vi "数据查询筛选弹框.vi"(8 "error in (no error)":errorcluster caption="错误输入（无错误）", 9 "是否初始化":enum16{"init", "keep"}(ring), 10 "database":string="database1.mdb", 11 "table":string(combo)="CODMn") -> (0 "error out":errorcluster caption="错误输出", 1 "确定输出":bool, 2 "显示项":string[](array[string]), 3 "condition":string)   [LabVIEW 2016]
uses:
  <vilib>/addons/database/Auxilliary.llb/DB Tools DataTypes.ctl
  <vilib>/picture/picture.llb/imagedata.ctl
  <vilib>/Utility/miscctls.llb/LVPointTypeDef.ctl
  <vilib>/addons/database/Connection.llb/DB Tools Open Connec (String).vi
  <vilib>/addons/database/Connection.llb/Conn Execute.vi
  <vilib>/addons/database/Recordset.llb/Rec Fetch Recordset Data (R).vi
  <vilib>/addons/database/Recordset.llb/Rec Destroy - Connection.vi
  <userlib>/_OpenG.lib/array/array.llb/Remove Duplicates from 1D Array (String)__ogtk.vi
  <vilib>/addons/database/_DB Variant To Data/Database Variant To Data.xnode
  <vilib>/addons/database/NI_Database_API.lvlib
panel:
  in  "背景图像":T1
  in  "实时分钟小时数据":enum32{"实时数据", "分钟数据", "小时数据"}(radio)
  in  "确定":bool
  out "自定义2single":cluster{"起始范围":string, "截止范围":string}
  out "自定义1single":cluster{"起始范围":string, "截止范围":string}
  out "自定义2筛选条件":string[](array[string])
  out "自定义1筛选条件":string[](array[string])
  in  "标签 2":string="从：\n\n\n至："
  in  "自定义数值结束 2":dbl
  in  "自定义数值起始 2":dbl
  in  "自定义结束时间 2":timestamp(xcontrol)
  in  "自定义起始时间 2":timestamp(xcontrol)
  in  "自定义 2":T2 caption="自定义"
  in  "下拉列表":string(xcontrol)
  in  "标签":string="从：\n\n\n至："
  in  "自定义数值结束":dbl
  in  "自定义数值起始":dbl
  in  "自定义结束时间":timestamp(xcontrol)
  in  "自定义起始时间":timestamp(xcontrol)
  in  "自定义":T2
  in  "下拉列表 2":string(xcontrol)
  out "type":T3[](array[typedef])
  out "所有测量模式":string[](array[string])
  out "数组":string[](array[string])
  out "columns":string[](array[string])
  in  "测量模式":T4
  in  "退出":bool
  in  "清空":bool
  in  "时间标识输入1":timestamp(xcontrol)
  in  "时间标识输入2":timestamp(xcontrol)
  # "时间"
  # "从："
  # "至："
  # "测试模式"
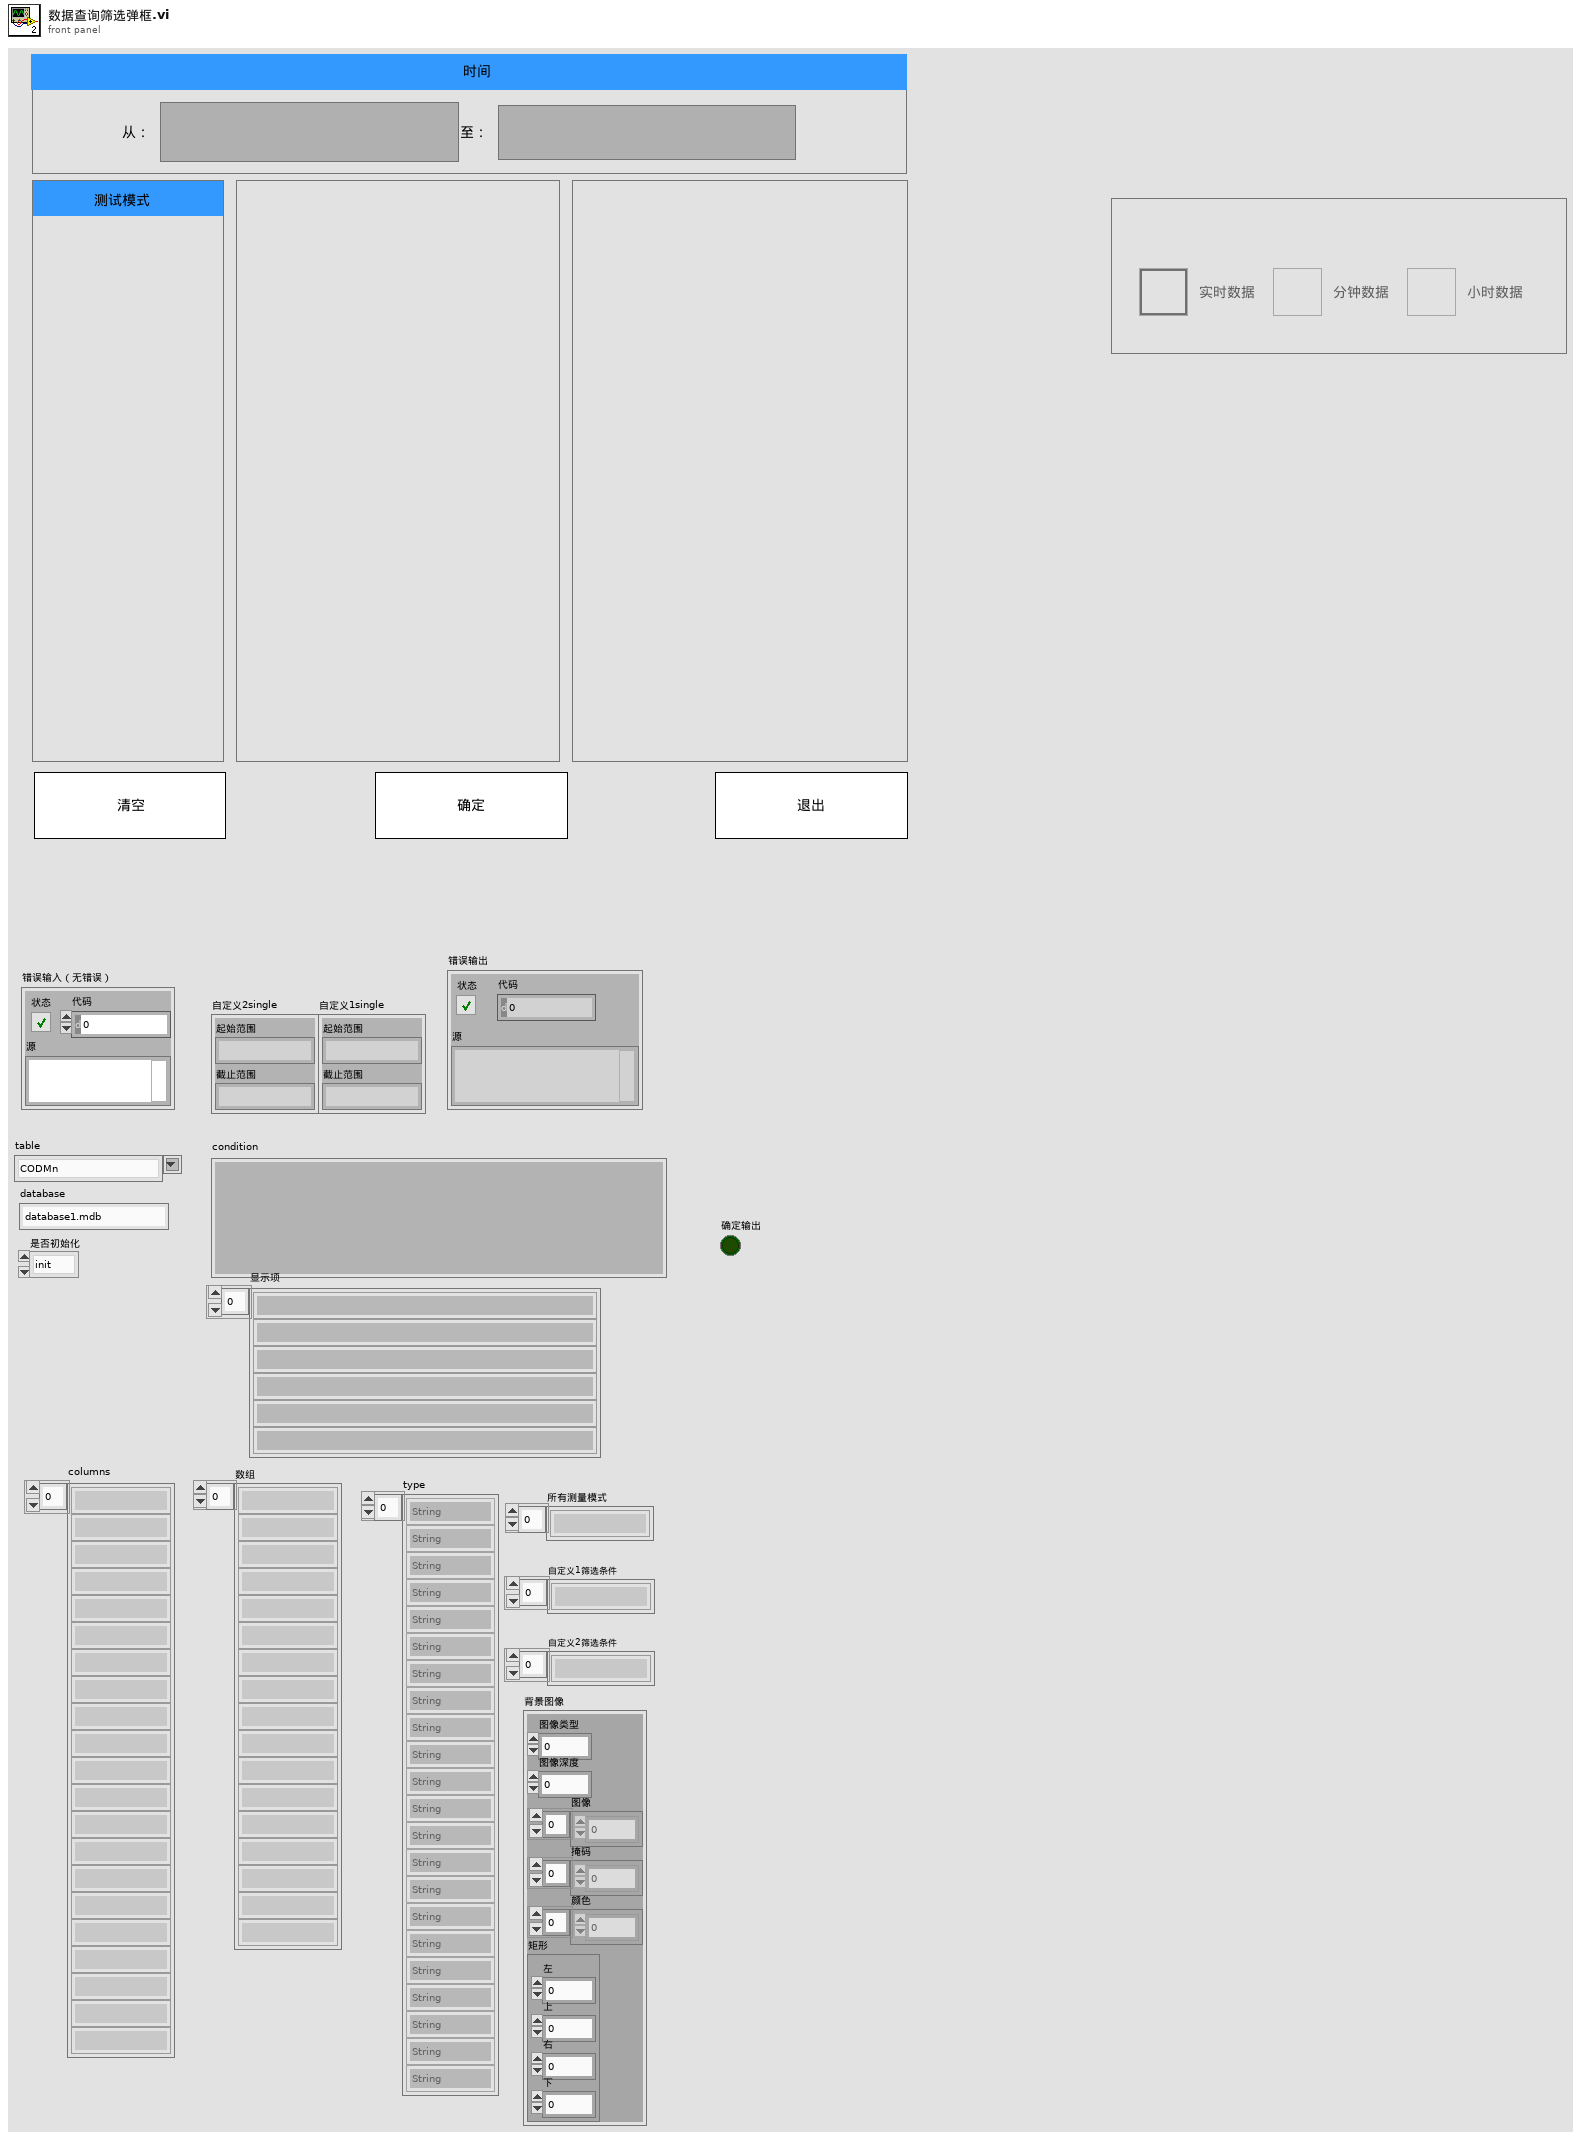
[diagram p1: front panel]
types:
  T1 = typedef "imagedata.ctl" = cluster{"image type":i32, "image depth":i32, "image":u8[], "mask":u8[], "colors":u32[], "Rectangle":cluster{"left":i16, "top":i16, "right":i16, "bottom":i16}}
  T2 = cluster{"DSADSA ":bool, "2":bool, "3":bool, "4":bool, "5":bool, "6":bool, "7":bool, "8":bool, "9":bool, "10":bool}
  T3 = typedef "NI_Database_API.lvlib/DB Tools DataTypes.ctl" = enum16{"String", "Long (I32)", "Single (SGL)", "Double (DBL)", "Date/Time", "Binary"}
  T4 = cluster{"水样测试":bool, "标样核查":bool, "零点核查":bool, "跨度核查":bool, "空白测试":bool, "平行样测试":bool, "加标回收":bool, "空白校准":bool, "标样校准":bool, "初始化清洗":bool}
  T5 = enum8{"Enabled", "Disabled", "Disabled and Grayed Out"}
  T6 = typedef "LVPointTypeDef.ctl" = cluster{"Horizontal":i16, "Vertical":i16}
  T7 = typedef "NI_Database_API.lvlib/Conn ObjectReference.ctl" = refnum<k1>
  T8 = cluster{"name":string, "database data type":T3, "defined size":i32}[]
  T9 = typedef "NI_Database_API.lvlib/Rec ObjectReference.ctl" = refnum<k1>
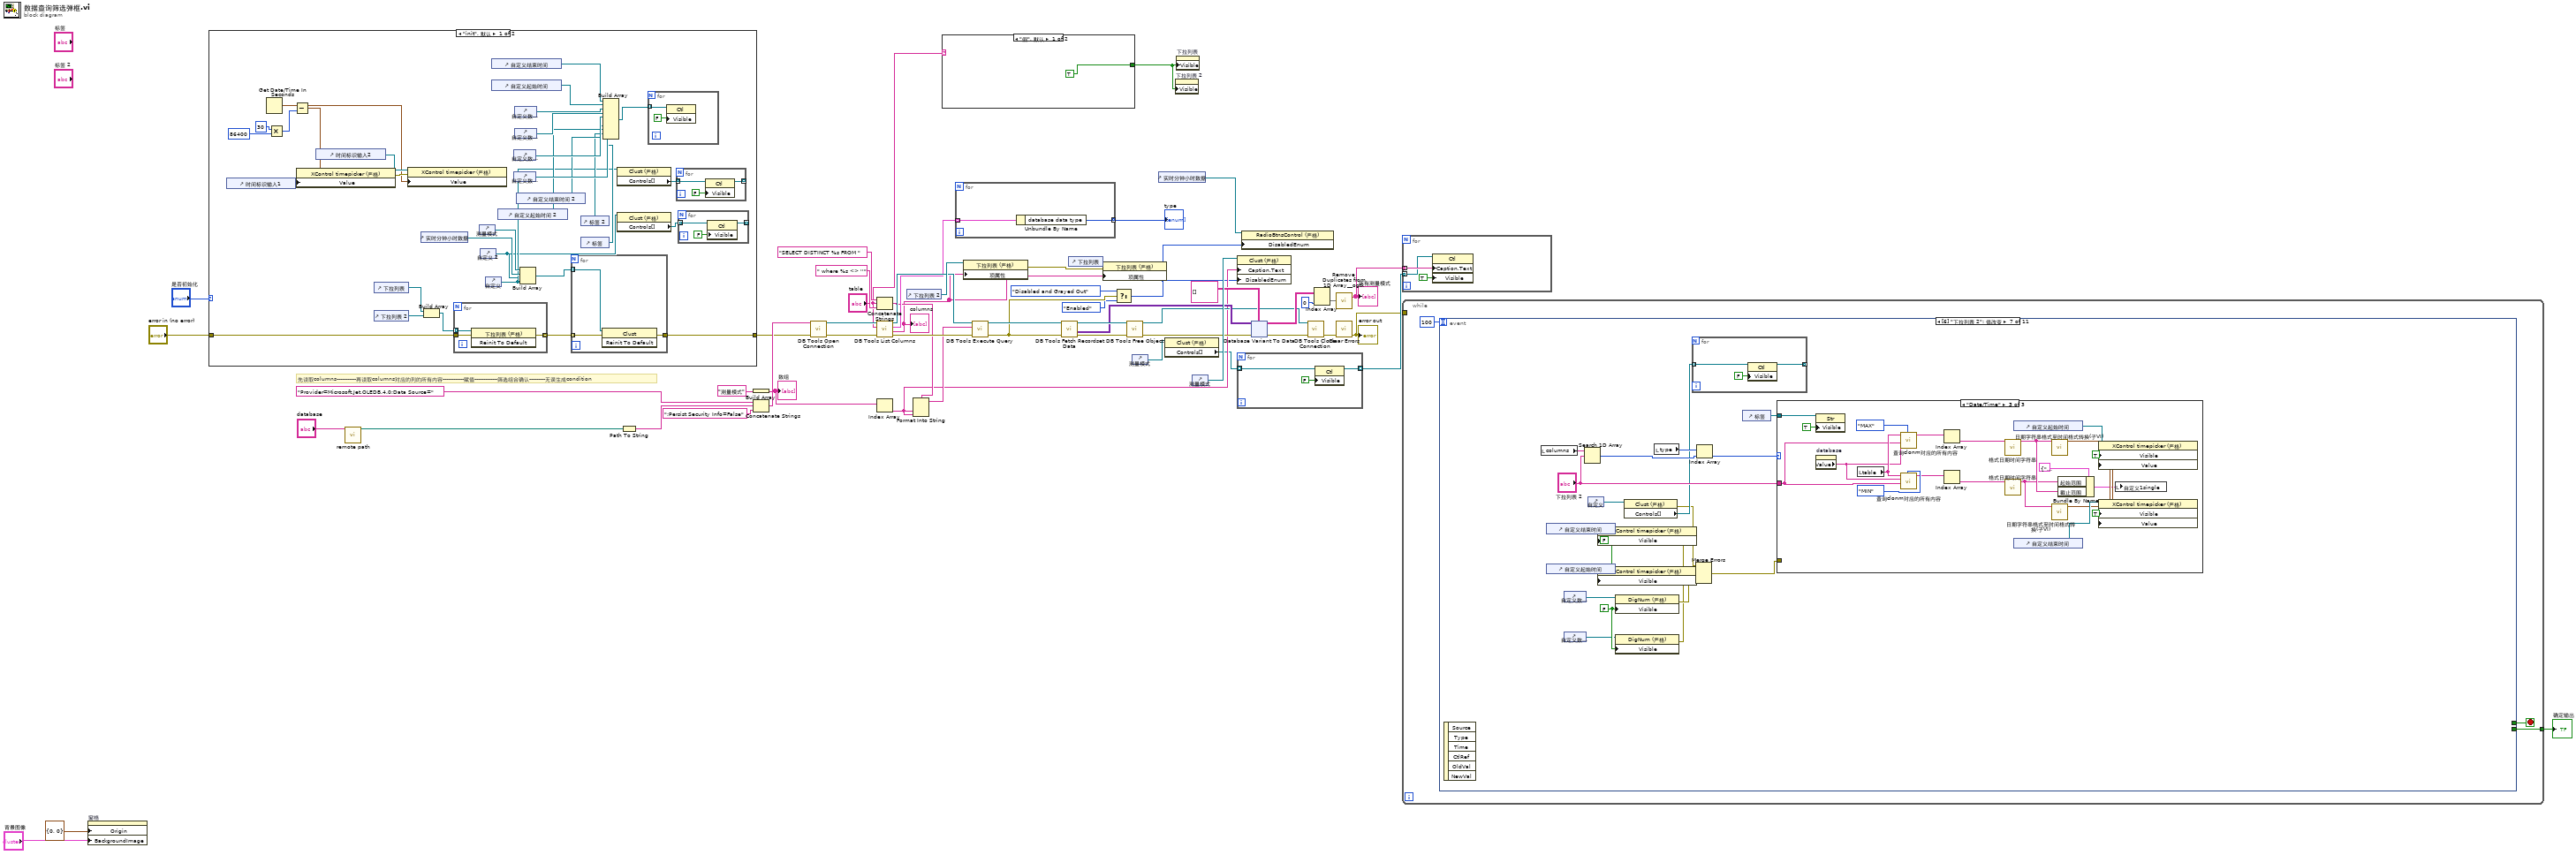
[diagram p0: block diagram]
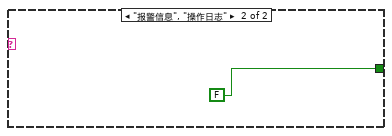
[diagram p2: hidden frame]
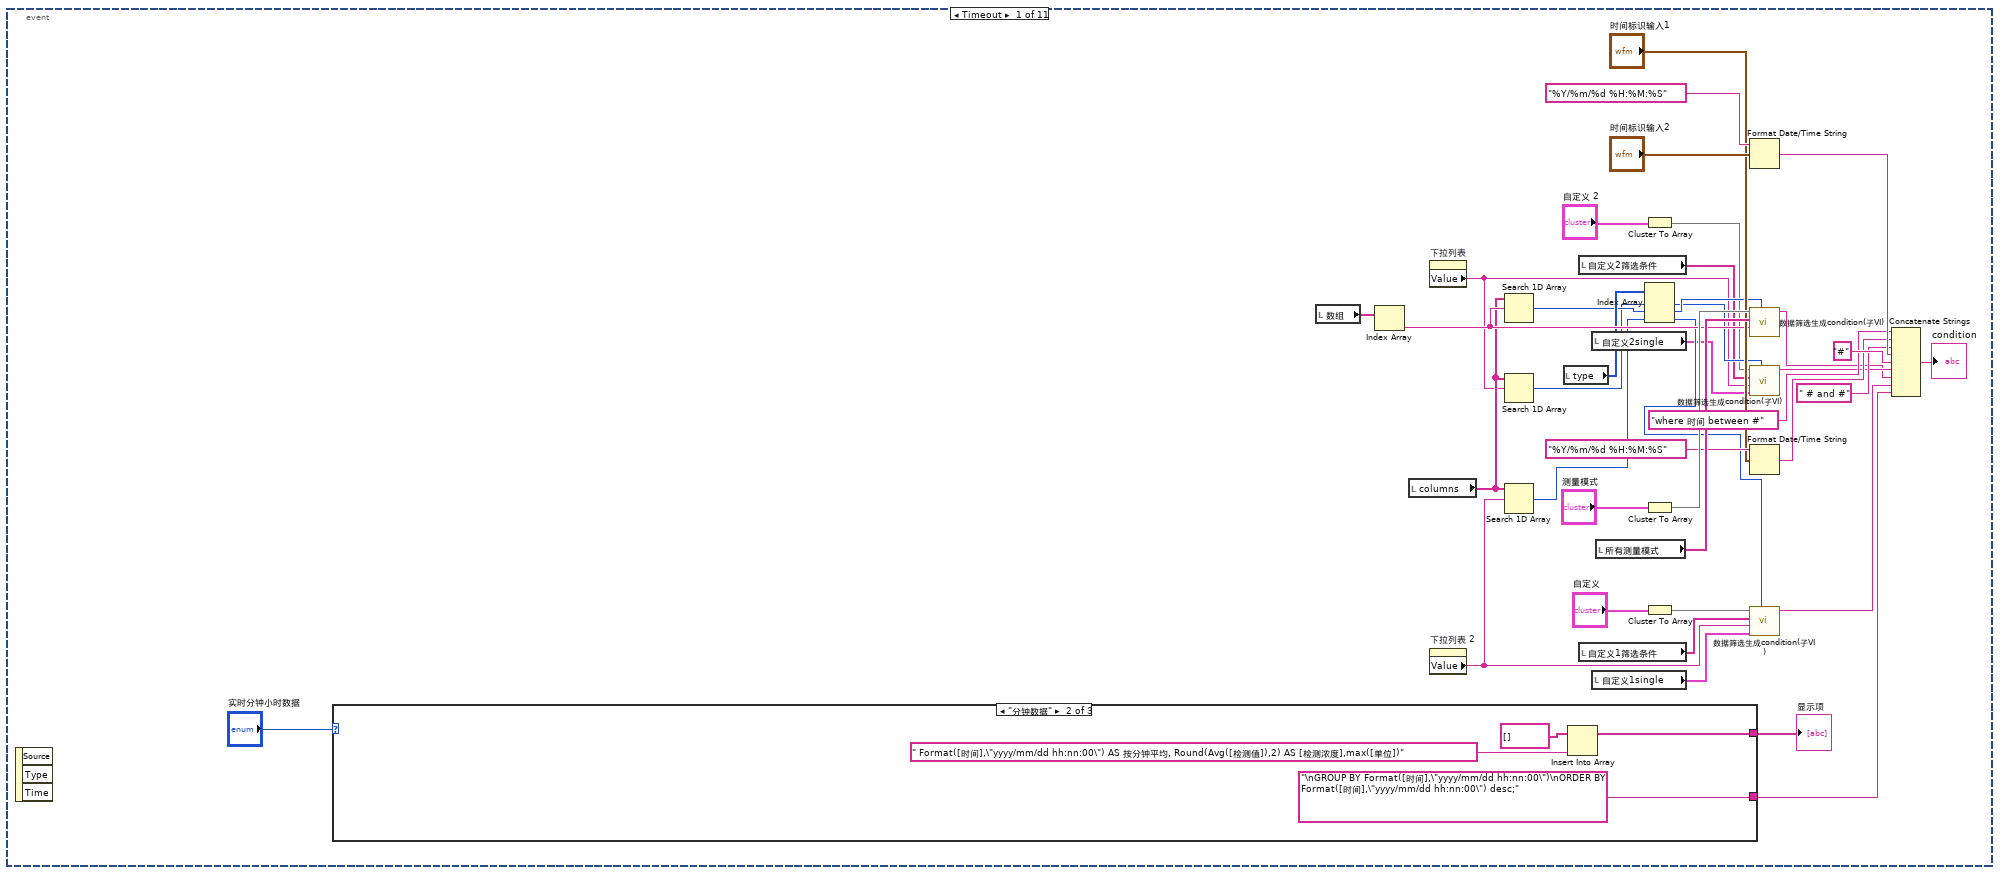
[diagram p4: hidden frame]
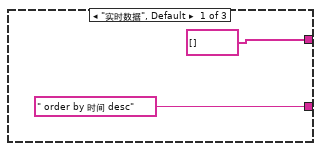
[diagram p5: hidden frame]
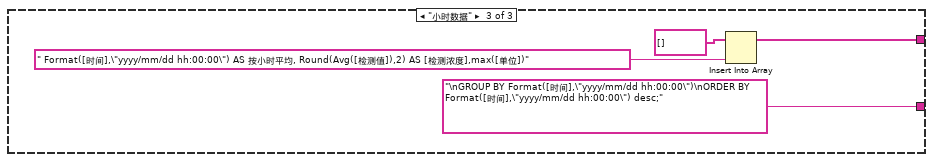
[diagram p6: hidden frame]
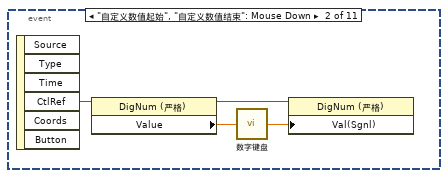
[diagram p7: hidden frame]
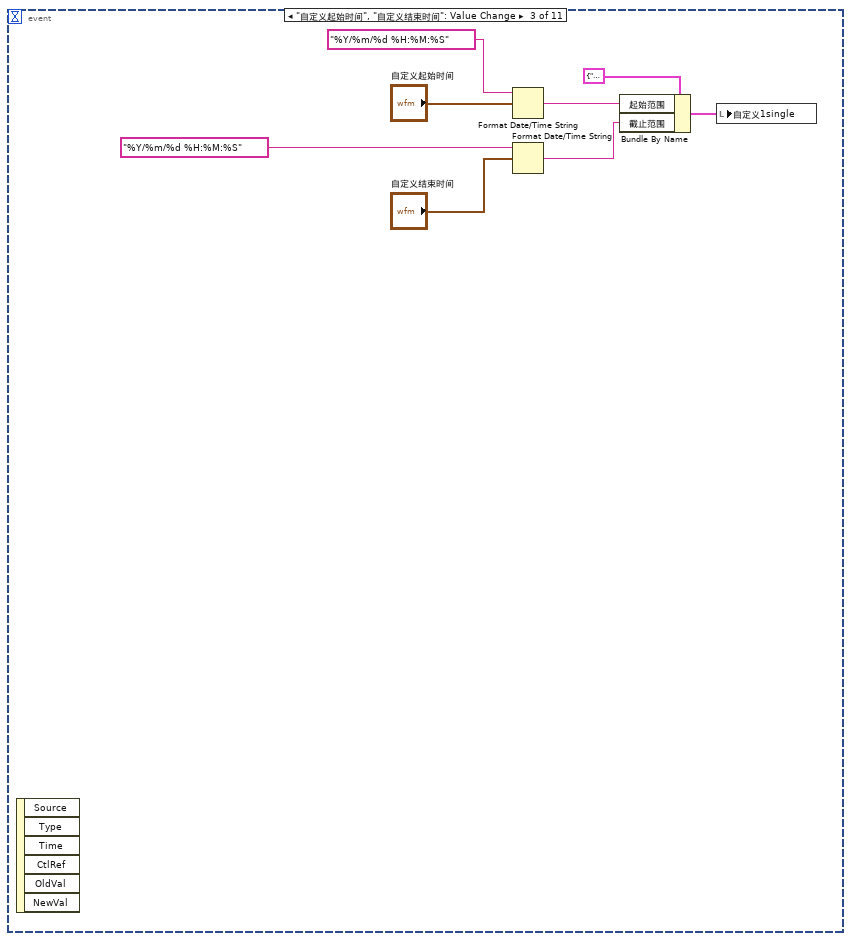
[diagram p8: hidden frame]
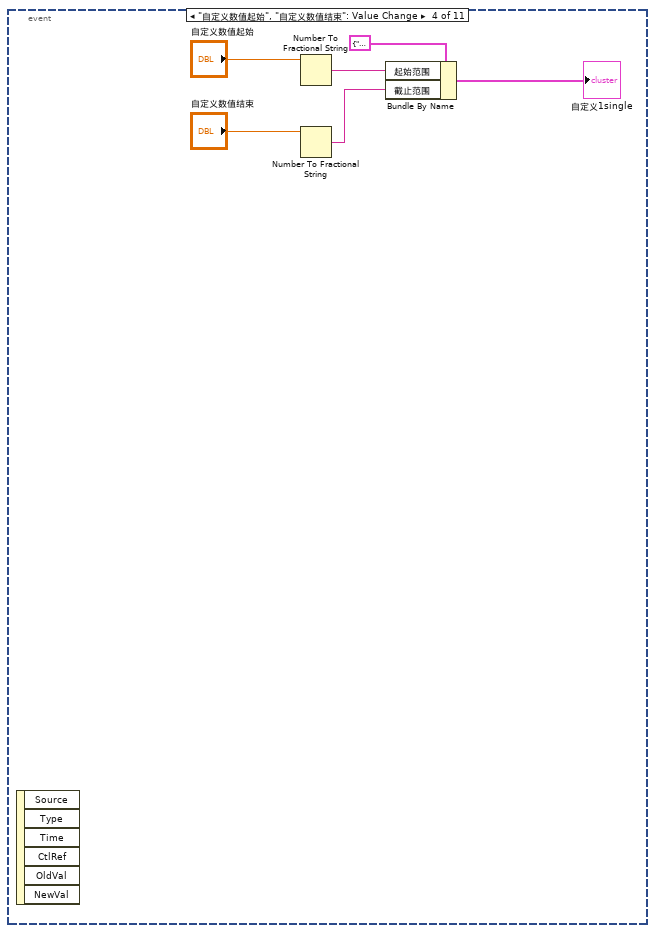
[diagram p9: hidden frame]
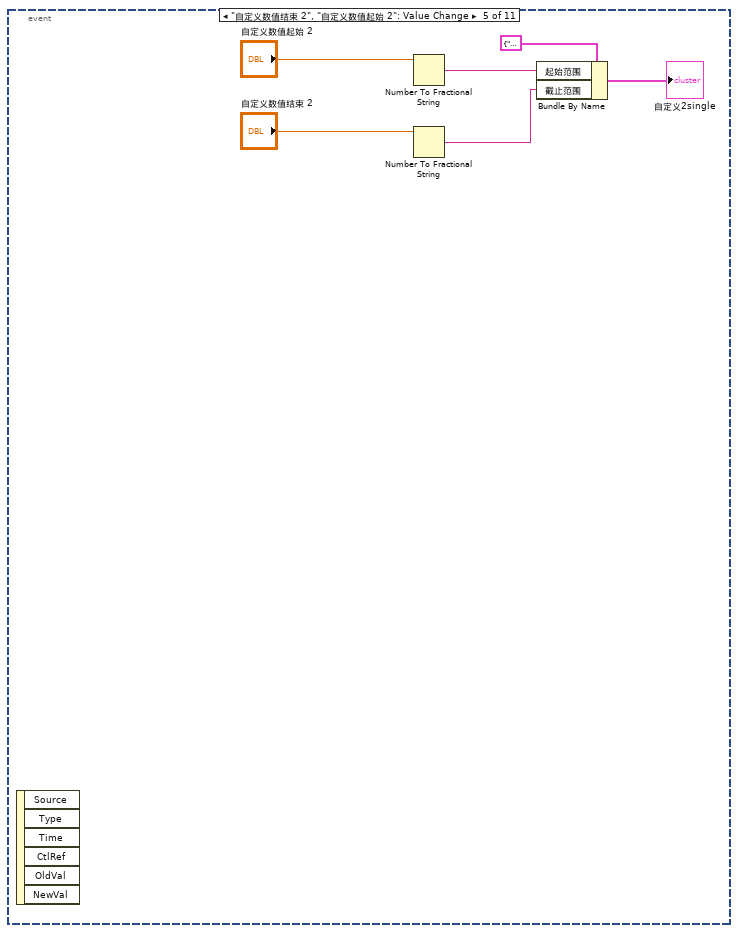
[diagram p10: hidden frame]
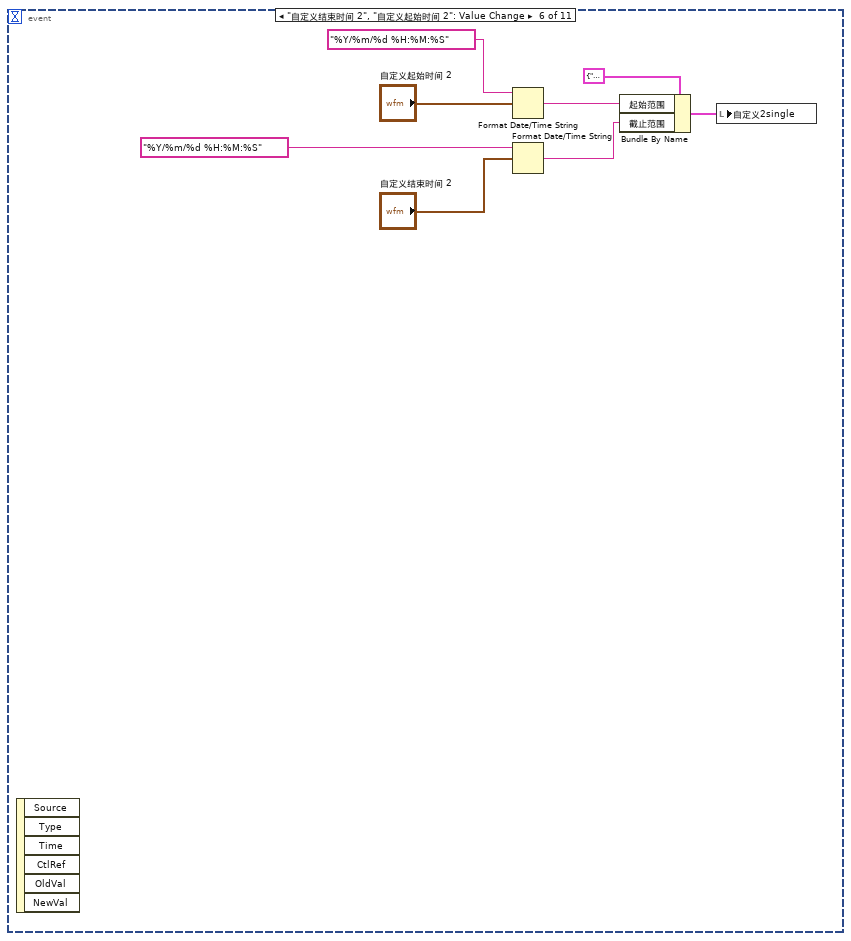
[diagram p11: hidden frame]
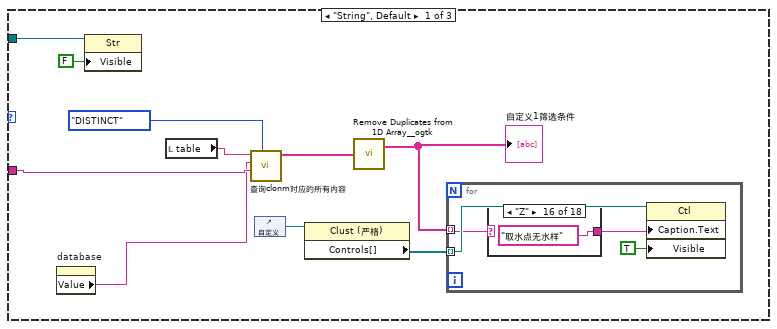
[diagram p12: hidden frame]
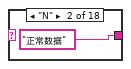
[diagram p14: hidden frame]
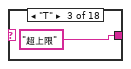
[diagram p15: hidden frame]
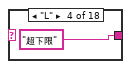
[diagram p16: hidden frame]
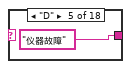
[diagram p17: hidden frame]
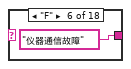
[diagram p18: hidden frame]
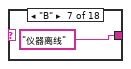
[diagram p19: hidden frame]
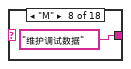
[diagram p20: hidden frame]
diagram:
  # "先读取columns-----------再读取columns对应的列的所有内容------------赋值-------------筛选组合确认---------无误生成condition"
  n1 = property on="窗格" class="Pane"("Origin"=T6 {"Horizontal"=0, "Vertical"=0} ("原点"), "BackgroundImage"="背景图像") -> ()  [unwired: 2 in, 2 out]
  n2 = case shown="\"init\", 默认" "是否初始化" {
    tunnel: "error in (no error)" -> [w64 w101]
    tunnel: [w83 w101] -> w11
    frame "init", Default {
      n3 = control-ref of="时间标识输入1"() -> (w66:refnum<vi>)
      n4 = Get Date/Time In Seconds() -> (seconds since 1Jan1904=w59:timestamp)
      n5 = Multiply(x=30, y=86400) -> (x*y=w78:i32)
      n6 = Subtract(x=w59, y=w78) -> (x-y=w82:timestamp)
      n7 = property class="XControl timepicker (严格)"(reference=w66, "Value"=w82) -> (error out=w81:errorcluster)  [unwired: 1 in, 1 out]
      n8 = control-ref of="时间标识输入2"() -> (w65:refnum<vi>)
      n9 = control-ref of="下拉列表"() -> (w62:refnum<vi>)
      n10 = control-ref of="下拉列表 2"() -> (w61:refnum<vi>)
      n11 = property class="XControl timepicker (严格)"(reference=w65, error in=w81, "Value"=w59) -> ()  [unwired: 2 out]
      n12 = control-ref of="实时分钟小时数据"() -> (w86:refnum<vi>)
      n13 = Build Array(w62, w61) -> (w60:refnum<vi>[])
      n14 = for {
        tunnel: w64 -> [w95]
        tunnel: [w94] -> w63 mode=indexing
        tunnel: w60 -> [w93] mode=indexing
        n15 = invoke class="下拉列表 (严格)" method="Reinit To Default"(reference=w93, error in=w95) -> (error out=w94:errorcluster)  [unwired: 1 in, 2 out]
      }
      n16 = control-ref of="测量模式"() -> (w84:refnum<vi>)
      n17 = control-ref of="自定义 2"() -> (w56:refnum<vi>)
      n18 = control-ref of="自定义"() -> (w58:refnum<vi>)
      n19 = control-ref of="自定义结束时间"() -> (w77:refnum<vi>)
      n20 = control-ref of="自定义起始时间"() -> (w76:refnum<vi>)
      n21 = control-ref of="自定义起始时间 2"() -> (w71:refnum<vi>)
      n22 = control-ref of="自定义数值结束 2"() -> (w73:refnum<vi>)
      n23 = control-ref of="自定义数值起始 2"() -> (w72:refnum<vi>)
      n24 = control-ref of="自定义数值结束"() -> (w75:refnum<vi>)
      n25 = control-ref of="自定义数值起始"() -> (w74:refnum<vi>)
      n26 = control-ref of="自定义结束时间 2"() -> (w70:refnum<vi>)
      n27 = Build Array(w84, w86, w56, w58) -> (w85:refnum<vi>[])
      n28 = for {
        tunnel: w85 -> [w100] mode=indexing
        tunnel: w63 -> [w99] mode=indexing
        tunnel: [w98] -> w83
        n29 = invoke class="Clust" method="Reinit To Default"(reference=w100, error in=w99) -> (error out=w98:errorcluster)  [unwired: 1 in, 2 out]
      }
      n30 = control-ref of="标签 2"() -> (w67:refnum<vi>)
      n31 = control-ref of="标签"() -> (w68:refnum<vi>)
      n32 = Build Array(w77, w76, w75, w74, w73, w72, w70, w71, w67, w68) -> (w69:refnum<vi>[])
      n33 = property class="Clust (严格)"(reference=w58) -> ("Controls[]"=w57:refnum<vi>[])  [unwired: 1 in, 2 out]
      n34 = property class="Clust (严格)"(reference=w56) -> ("Controls[]"=w55:refnum<vi>[])  [unwired: 1 in, 2 out]
      n35 = for {
        tunnel: w69 -> [w97] mode=indexing
        n36 = property class="Ctl"(reference=w97, "Visible"=FALSE ("可见")) -> ()  [unwired: 1 in, 2 out]
      }
      n37 = for {
        tunnel: w57 -> [w92] mode=indexing
        tunnel: [w90] -> _ mode=indexing
        n38 = property class="Ctl"(reference=w92, "Visible"=FALSE ("可见")) -> (reference out=w90:refnum<vi>)  [unwired: 1 in, 1 out]
      }
      n39 = for {
        tunnel: w55 -> [w89] mode=indexing
        tunnel: [w87] -> _ mode=indexing
        n40 = property class="Ctl"(reference=w89, "Visible"=FALSE ("可见")) -> (reference out=w87:refnum<vi>)  [unwired: 1 in, 1 out]
      }
    }
    frame "keep" {
    }
  }
  n41 = call "remote path.vi"("database"="database") -> ("appended path"=w49:path)  [unwired: 10 in]
  n42 = Path To String(path=w49) -> (string=w51:string)
  n43 = Build Array("测量模式" ("Element Data")) -> (w14:string[])
  "数组" <- w14
  n44 = Concatenate Strings("Provider=Microsoft.Jet.OLEDB.4.0;Data Source=", w51, ";Persist Security Info=False") -> (w50:string)
  n45 = call-poly <vilib>:"DB Tools Open Connection.vi"("error in (no error)"=w11, "connection information"=w50) -> ("error out"=w47:errorcluster, "connection reference"=w48:T7)  [unwired: 6 in]
  n46 = Concatenate Strings("SELECT DISTINCT %s FROM " ("字符串"), "table", " where %s <> ''" ("字符串")) -> (w24:string)
  n47 = call <vilib>:"DB Tools List Columns.vi"("error in (no error)"=w47, "table"="table", "connection reference"=w48) -> ("error out"=w41:errorcluster, "columns"=w4:string[], "column information"=w28:T8, "connection reference out"=w29:T7)  [unwired: 1 in]
  "columns" <- w4
  n48 = Index Array(array=w14) -> (element=w23:string)  [unwired: 1 in]
  n49 = control-ref of="下拉列表 2"() -> (w30:refnum<vi>)
  n50 = Format Into String(format string=w24, w23, w23) -> (resulting string=w40:string)  [unwired: 2 in, 1 out]
  n51 = case shown="\"假\", 默认" "table" {
    tunnel: [TRUE FALSE] -> w1
    frame "假", Default {
    }
    frame "报警信息", "操作日志" {
    }
  }
  n52 = for {
    tunnel: w28 -> [w105] mode=indexing
    tunnel: [w104] -> w27 mode=indexing
    n53 = Unbundle By Name(w105) -> ("database data type"=w104:T3)
  }
  "type" <- w27
  n54 = property class="下拉列表 (严格)"(reference=w30, "项属性"=w4) -> (error out=w10:errorcluster)  [unwired: 1 in, 1 out]
  n55 = call-poly <vilib>:"DB Tools Execute Query.vi"("error in (no error)"=w41, "SQL query"=w40, "connection reference"=w29) -> ("error out"=w22:errorcluster, "recordset reference"=w44:T9)  [unwired: 5 in]
  n56 = call-poly <vilib>:"DB Tools Fetch Recordset Data.vi"("error in (no error)"=w22, "recordset reference"=w44) -> ("error out"=w43:errorcluster, "recordset data"=w36:variant[][], "recordset reference out"=w42:T9)  [unwired: 3 in]
  n57 = control-ref of="下拉列表"() -> (w19:refnum<vi>)
  n58 = property class="下拉列表 (严格)"(reference=w19, error in=w10, "项属性"=w4) -> ()  [unwired: 2 out]
  n59 = Select(t=T5."Disabled and Grayed Out" ("禁用"), s=w22, f=T5."Enabled" ("禁用")) -> (s? t:f=w6:T5)
  n60 = call-poly <vilib>:"DB Tools Free Object.vi"("error in (no error)"=w43, "recordset reference"=w42) -> ("error out"=w35:errorcluster, "connection reference"=w34:T7)  [unwired: 8 in]
  n61 = control-ref of="测量模式"() -> (w54:refnum<vi>)
  n62 = control-ref of="实时分钟小时数据"() -> (w7:refnum<vi>)
  n63 = property class="Clust (严格)"(reference=w54) -> ("Controls[]"=w18:refnum<vi>[])  [unwired: 1 in, 2 out]
  n64 = property on="下拉列表 2" class="下拉列表 (严格)"("Visible"=w1) -> ()  [unwired: 2 in, 2 out]
  n65 = property on="下拉列表" class="下拉列表 (严格)"("Visible"=w1) -> ()  [unwired: 2 in, 2 out]
  n66 = control-ref of="测量模式"() -> (w45:refnum<vi>)
  n67 = property class="Clust (严格)"(reference=w45, "Caption.Text"=w23, "DisabledEnum"=w6) -> ()  [unwired: 1 in, 2 out]
  n68 = for {
    tunnel: w18 -> [w108] mode=indexing
    tunnel: [w106] -> w17 mode=indexing
    n69 = property class="Ctl"(reference=w108, "Visible"=FALSE ("可见")) -> (reference out=w106:refnum<vi>)  [unwired: 1 in, 1 out]
  }
  n70 = property class="RadioBtnsControl (严格)"(reference=w7, "DisabledEnum"=w6) -> ()  [unwired: 1 in, 2 out]
  n71 = xnode "Database Variant To Data"("database variant"=w36, "error in (no error)"=w35, "type"=string[][] []) -> ("data"=w37:string[][], "error out"=w38:errorcluster)
  n72 = call <vilib>:"DB Tools Close Connection.vi"("error in (no error)"=w38, "connection reference"=w34) -> ("error out"=w13:errorcluster)  [unwired: 5 in]
  n73 = Index Array(array=w37, index (col)=0 ("禁用的索引 (列)")) -> (element=w32:string[])  [unwired: 1 in]
  n74 = call-poly <userlib>:"Remove Duplicates from 1D Array__ogtk.vi"("Input Array"=w32) -> ("Output Array"=w16:string[])  [unwired: 1 out]
  "所有测量模式" <- w16
  n75 = call <vilib>:"Clear Errors.vi"("error in (no error)"=w13) -> ("error out"=w8:errorcluster)  [unwired: 5 in, 1 out]
  "error out" <- w8
  n76 = for {
    tunnel: w16 -> [w111] mode=indexing
    tunnel: w17 -> [w109] mode=indexing
    n77 = property class="Ctl"(reference=w109, "Caption.Text"=w111, "Visible"=TRUE ("可见")) -> ()  [unwired: 1 in, 2 out]
  }
  n78 = while {
    tunnel: [w112] -> w15
    tunnel: w8 -> [_]
    stop <- w114 stop-if-true
    n79 = event shown="[6] \"下拉列表 2\": 值改变" {
      selector: _ -> [_ _ _ _ _ _ _ _ _ _ _]
      dyn-events: _ -> [_ _ _ _ _ _ _ _ _ _ _]
      timeout: 100 -> [_ _ _ _ _ _ _ _ _ _ _]
      tunnel: [_ _ _ _ _ _ _ _ _ w394 TRUE] -> w114
      tunnel: [_ _ _ _ _ _ _ _ _ w394 _] -> w112
      event Timeout {
        n80 = event-data() -> ()  [unwired: 1 in, 3 out]
        n81 = case shown="\"分钟数据\"" "实时分钟小时数据" {
          tunnel: [string[] [] ("显示项") w156 w160] -> w115
          tunnel: [" order by 时间 desc" ("字符串") "\nGROUP BY Format([时间],\"yyyy/mm/dd hh:nn:00\")\nORDER BY Format([时间],\"yyyy/mm/dd hh:nn:00\") desc;" ("字符串") "\nGROUP BY Format([时间],\"yyyy/mm/dd hh:00:00\")\nORDER BY Format([时间],\"yyyy/mm/dd hh:00:00\") desc;" ("字符串")] -> w116
          frame "实时数据", Default {
          }
          frame "分钟数据" {
            n82 = Insert Into Array(array=string[] [] ("显示项"), new element=" Format([时间],\"yyyy/mm/dd hh:nn:00\") AS 按分钟平均, Round(Avg([检测值]),2) AS [检测浓度],max([单位])" ("新元素/子数组")) -> (w156:string[])  [unwired: 1 in]
          }
          frame "小时数据" {
            n83 = Insert Into Array(array=string[] [] ("显示项"), new element=" Format([时间],\"yyyy/mm/dd hh:00:00\") AS 按小时平均, Round(Avg([检测值]),2) AS [检测浓度],max([单位])" ("新元素/子数组")) -> (w160:string[])  [unwired: 1 in]
          }
        }
        "显示项" <- w115
        n84 = local read "数组"() -> (w153:string[])
        n85 = Index Array(array=w153) -> (element=w139:string)  [unwired: 1 in]
        n86 = local read "columns"() -> (w133:string[])
        n87 = property on="下拉列表" class="下拉列表 (严格)"() -> ("Value"=w124:string)  [unwired: 2 in, 2 out]
        n88 = property on="下拉列表 2" class="下拉列表 (严格)"() -> ("Value"=w123:string)  [unwired: 2 in, 2 out]
        n89 = Search 1D Array(1D array=w133, element=w139) -> (index of element=w137:i32)  [unwired: 1 in]
        n90 = Search 1D Array(1D array=w133, element=w124) -> (index of element=w132:i32)  [unwired: 1 in]
        n91 = Search 1D Array(1D array=w133, element=w123) -> (index of element=w135:i32)  [unwired: 1 in]
        n92 = local read "type"() -> (w138:T3[])
        n93 = local read "自定义2筛选条件"() -> (w121:string[])
        n94 = local read "自定义1筛选条件"() -> (w122:string[])
        n95 = local read "自定义2single"() -> (w119:cluster{"起始范围":string, "截止范围":string})
        n96 = local read "自定义1single"() -> (w118:cluster{"起始范围":string, "截止范围":string})
        n97 = local read "所有测量模式"() -> (w152:string[])
        n98 = Cluster To Array(cluster="自定义 2") -> (array=w130:bool[])
        n99 = Index Array(array=w138, index #1=w132, index #2=w137, index #3=w135) -> (element #1=w131:T3, element #2=w136:T3, element #3=w134:T3)
        n100 = Cluster To Array(cluster="测量模式") -> (array=w151:bool[])
        n101 = Cluster To Array(cluster="自定义") -> (array=w120:bool[])
        n102 = Format Date/Time String(time format string (%c)="%Y/%m/%d %H:%M:%S" ("时间格式字符串(%c)"), seconds (now)="时间标识输入2") -> (date/time string=w148:string)  [unwired: 1 in]
        n103 = call "数据筛选生成condition(子VI).vi"("database data type"=w136, "段名"=w139, "筛选内容"=w152, "簇转数组"=w151) -> ("condition"=w128:string)  [unwired: 7 in]
        n104 = call "数据筛选生成condition(子VI).vi"("database data type"=w131, "Single"=w119, "段名"=w124, "筛选内容"=w121, "簇转数组"=w130) -> ("condition"=w129:string)  [unwired: 6 in]
        n105 = Format Date/Time String(time format string (%c)="%Y/%m/%d %H:%M:%S" ("时间格式字符串(%c)"), seconds (now)="时间标识输入1") -> (date/time string=w146:string)  [unwired: 1 in]
        n106 = call "数据筛选生成condition(子VI).vi"("database data type"=w134, "Single"=w118, "段名"=w123, "筛选内容"=w122, "簇转数组"=w120) -> ("condition"=w127:string)  [unwired: 6 in]
        n107 = Concatenate Strings("where 时间 between #", w146, " # and #" ("condition"), w148, "#" ("condition"), w129, w128, w127, w116) -> (→"condition":string)
      }
      event "自定义数值起始", "自定义数值结束": Mouse Down {
        n108 = event-data() -> ("CtlRef"=w167:refnum<vi>)  [unwired: 1 in, 5 out]
        n109 = property class="DigNum (严格)"(reference=w167) -> (reference out=w165:refnum<vi>, "Value"=w166:dbl)  [unwired: 1 in, 1 out]
        n110 = call "数字键盘.vi"("OldNumber"=w166) -> ("NewNumber"=w164:sgl)
        n111 = property class="DigNum (严格)"(reference=w165, "Val(Sgnl)"=w164) -> ()  [unwired: 1 in, 2 out]
      }
      event "自定义起始时间", "自定义结束时间": Value Change {
        n112 = event-data() -> ()  [unwired: 1 in, 6 out]
        n113 = Format Date/Time String(time format string (%c)="%Y/%m/%d %H:%M:%S" ("时间格式字符串(%c)"), seconds (now)="自定义起始时间") -> (date/time string=w174:string)  [unwired: 1 in]
        n114 = Format Date/Time String(time format string (%c)="%Y/%m/%d %H:%M:%S" ("时间格式字符串(%c)"), seconds (now)="自定义结束时间") -> (date/time string=w175:string)  [unwired: 1 in]
        n115 = Bundle By Name(cluster=cluster{"起始范围":string, "截止范围":string} {"起始范围"="2", "截止范围"="5"} ("Single"), "起始范围"=w174, "截止范围"=w175) -> (w168:cluster{"起始范围":string, "截止范围":string})
        n116 = local write "自定义1single"(w168) -> ()
      }
      event "自定义数值起始", "自定义数值结束": Value Change {
        n117 = event-data() -> ()  [unwired: 1 in, 6 out]
        n118 = Number To Fractional String(number="自定义数值起始") -> (F-format string=w180:string)  [unwired: 3 in]
        n119 = Number To Fractional String(number="自定义数值结束") -> (F-format string=w181:string)  [unwired: 3 in]
        n120 = Bundle By Name(cluster=cluster{"起始范围":string, "截止范围":string} {"起始范围"="2", "截止范围"="5"} ("Single"), "起始范围"=w180, "截止范围"=w181) -> (→"自定义1single":cluster{"起始范围":string, "截止范围":string})
      }
      event "自定义数值结束 2", "自定义数值起始 2": Value Change {
        n121 = event-data() -> ()  [unwired: 1 in, 6 out]
        n122 = Number To Fractional String(number="自定义数值起始 2") -> (F-format string=w184:string)  [unwired: 3 in]
        n123 = Number To Fractional String(number="自定义数值结束 2") -> (F-format string=w183:string)  [unwired: 3 in]
        n124 = Bundle By Name(cluster=cluster{"起始范围":string, "截止范围":string} {"起始范围"="2", "截止范围"="5"} ("Single"), "起始范围"=w184, "截止范围"=w183) -> (→"自定义2single":cluster{"起始范围":string, "截止范围":string})
      }
      event "自定义结束时间 2", "自定义起始时间 2": Value Change {
        n125 = event-data() -> ()  [unwired: 1 in, 6 out]
        n126 = Format Date/Time String(time format string (%c)="%Y/%m/%d %H:%M:%S" ("时间格式字符串(%c)"), seconds (now)="自定义起始时间 2") -> (date/time string=w193:string)  [unwired: 1 in]
        n127 = Format Date/Time String(time format string (%c)="%Y/%m/%d %H:%M:%S" ("时间格式字符串(%c)"), seconds (now)="自定义结束时间 2") -> (date/time string=w194:string)  [unwired: 1 in]
        n128 = Bundle By Name(cluster=cluster{"起始范围":string, "截止范围":string} {"起始范围"="2", "截止范围"="5"} ("Single"), "起始范围"=w193, "截止范围"=w194) -> (w195:cluster{"起始范围":string, "截止范围":string})
        n129 = local write "自定义2single"(w195) -> ()
      }
      event "下拉列表 2": Value Change {
        w206 = FALSE ("可见")
        w196 = FALSE ("可见")
        n130 = event-data() -> ()  [unwired: 1 in, 6 out]
        n131 = local read "columns"() -> (w213:string[])
        n132 = control-ref of="自定义结束时间"() -> (w208:refnum<vi>)
        n133 = control-ref of="自定义起始时间"() -> (w207:refnum<vi>)
        n134 = control-ref of="自定义数值结束"() -> (w205:refnum<vi>)
        n135 = control-ref of="自定义数值起始"() -> (w198:refnum<vi>)
        n136 = Search 1D Array(1D array=w213, element="下拉列表 2") -> (index of element=w215:i32)  [unwired: 1 in]
        n137 = control-ref of="自定义"() -> (w210:refnum<vi>)
        n138 = property class="XControl timepicker (严格)"(reference=w208, "Visible"=w196) -> (error out=w203:errorcluster)  [unwired: 1 in, 1 out]
        n139 = property class="XControl timepicker (严格)"(reference=w207, "Visible"=w196) -> (error out=w202:errorcluster)  [unwired: 1 in, 1 out]
        n140 = property class="DigNum (严格)"(reference=w205, "Visible"=w206) -> (error out=w201:errorcluster)  [unwired: 1 in, 1 out]
        n141 = property class="DigNum (严格)"(reference=w198, "Visible"=w206) -> (error out=w200:errorcluster)  [unwired: 1 in, 1 out]
        n142 = property class="Clust (严格)"(reference=w210) -> (error out=w204:errorcluster, "Controls[]"=w209:refnum<vi>[])  [unwired: 1 in, 1 out]
        n143 = local read "type"() -> (w214:T3[])
        n144 = for {
          tunnel: w209 -> [w218] mode=indexing
          tunnel: [w216] -> _ mode=indexing
          n145 = property class="Ctl"(reference=w218, "Visible"=FALSE ("可见")) -> (reference out=w216:refnum<vi>)  [unwired: 1 in, 1 out]
        }
        n146 = Merge Errors(w204, w203, w202, w201, w200) -> (w199:errorcluster)
        n147 = Index Array(array=w214, index=w215) -> (element=w211:T3)
        n148 = control-ref of="标签"() -> (w197:refnum<vi>)
        n149 = case shown="\"Date/Time\"" w211 {
          tunnel: "下拉列表 2" -> [w227 w259 w280]
          tunnel: w199 -> [_ _ _]
          tunnel: w197 -> [w222 w264 w284]
          frame "String", Default {
            n150 = property on="database" class="Str"() -> ("Value"=w219:string)  [unwired: 2 in, 2 out]
            n151 = property class="Str"(reference=w222, "Visible"=FALSE ("可见")) -> ()  [unwired: 1 in, 2 out]
            n152 = local read "table"() -> (w228:string)
            n153 = call "查询clonm对应的所有内容.vi"("条件"=enum16{"DISTINCT", "MIN", "MAX"}."DISTINCT", "组合框"=w227, "database"=w219, "table"=w228) -> ("输出数组"=w226:string[])  [unwired: 6 in, 1 out]
            n154 = control-ref of="自定义"() -> (w224:refnum<vi>)
            n155 = property class="Clust (严格)"(reference=w224) -> ("Controls[]"=w223:refnum<vi>[])  [unwired: 1 in, 2 out]
            n156 = call-poly <userlib>:"Remove Duplicates from 1D Array__ogtk.vi"("Input Array"=w226) -> ("Output Array"=w225:string[])  [unwired: 1 out]
            "自定义1筛选条件" <- w225
            n157 = for {
              tunnel: w225 -> [w229] mode=indexing
              tunnel: w223 -> [w231] mode=indexing
              n158 = case shown="\"Z\"" w229 {
                selector: w229 -> [w233 _ _ _ _ _ _ _ _ _ _ _ _ _ _ _ _ _]
                tunnel: [w233 "正常数据" "超上限" "超下限" "仪器故障" "仪器通信故障" "仪器离线" "维护调试数据" "缺试剂" "缺纯水" "缺水样" "缺标液" "加标回收" "平行样测试" "电源故障" "取水点无水样" "手工输入数据" "手动测试数据"] -> w230
                frame Default {
                }
                frame "N" {
                }
                frame "T" {
                }
                frame "L" {
                }
                frame "D" {
                }
                frame "F" {
                }
                frame "B" {
                }
                frame "M" {
                }
                frame "lr" {
                }
                frame "lp" {
                }
                frame "lw" {
                }
                frame "ls" {
                }
                frame "ra" {
                }
                frame "pt" {
                }
                frame "P" {
                }
                frame "Z" {
                }
                frame "S" {
                }
                frame "hd" {
                }
              }
              n159 = property class="Ctl"(reference=w231, "Caption.Text"=w230, "Visible"=TRUE ("可见")) -> ()  [unwired: 1 in, 2 out]
            }
          }
          frame "Long (I32)".."Double (DBL)" {
            w266 = TRUE ("可见")
            n160 = property on="database" class="Str"() -> ("Value"=w251:string)  [unwired: 2 in, 2 out]
            n161 = property class="Str"(reference=w264, "Visible"=TRUE ("可见")) -> ()  [unwired: 1 in, 2 out]
            n162 = local read "table"() -> (w260:string)
            n163 = call "查询clonm对应的所有内容.vi"("条件"=enum16{"DISTINCT", "MIN", "MAX"}."MAX", "组合框"=w259, "database"=w251, "table"=w260) -> ("输出数组"=w258:string[])  [unwired: 6 in, 1 out]
            n164 = call "查询clonm对应的所有内容.vi"("条件"=enum16{"DISTINCT", "MIN", "MAX"}."MIN", "组合框"=w259, "database"=w251, "table"=w260) -> ("输出数组"=w262:string[])  [unwired: 6 in, 1 out]
            n165 = Index Array(array=w258) -> (element=w253:string)  [unwired: 1 in]
            n166 = Index Array(array=w262) -> (element=w252:string)  [unwired: 1 in]
            n167 = control-ref of="自定义数值结束"() -> (w267:refnum<vi>)
            n168 = control-ref of="自定义数值起始"() -> (w268:refnum<vi>)
            n169 = Fract/Exp String To Number(string=w253) -> (number=w256:dbl)  [unwired: 3 in, 1 out]
            n170 = Fract/Exp String To Number(string=w252) -> (number=w257:dbl)  [unwired: 3 in, 1 out]
            n171 = Bundle By Name(cluster=cluster{"起始范围":string, "截止范围":string} {"起始范围"="2", "截止范围"="5"} ("Single"), "起始范围"=w252, "截止范围"=w253) -> (w254:cluster{"起始范围":string, "截止范围":string})
            n172 = property class="DigNum (严格)"(reference=w267, "Visible"=w266, "Value"=w256) -> ()  [unwired: 1 in, 2 out]
            n173 = property class="DigNum (严格)"(reference=w268, "Visible"=w266, "Value"=w257) -> ()  [unwired: 1 in, 2 out]
            n174 = local write "自定义1single"(w254) -> ()
          }
          frame "Date/Time" {
            n175 = property class="Str"(reference=w284, "Visible"=TRUE ("可见")) -> ()  [unwired: 1 in, 2 out]
            n176 = property on="database" class="Str"() -> ("Value"=w269:string)  [unwired: 2 in, 2 out]
            n177 = local read "table"() -> (w281:string)
            n178 = call "查询clonm对应的所有内容.vi"("条件"=enum16{"DISTINCT", "MIN", "MAX"}."MAX", "组合框"=w280, "database"=w269, "table"=w281) -> ("输出数组"=w279:string[])  [unwired: 6 in, 1 out]
            n179 = call "查询clonm对应的所有内容.vi"("条件"=enum16{"DISTINCT", "MIN", "MAX"}."MIN", "组合框"=w280, "database"=w269, "table"=w281) -> ("输出数组"=w274:string[])  [unwired: 6 in, 1 out]
            n180 = Index Array(array=w279) -> (element=w273:string)  [unwired: 1 in]
            n181 = Index Array(array=w274) -> (element=w271:string)  [unwired: 1 in]
            n182 = call "格式日期时间字符串.vi"("data[0]"=w273) -> ("日期/时间字符串"=w272:string)  [unwired: 10 in]
            n183 = call "格式日期时间字符串.vi"("data[0]"=w271) -> ("日期/时间字符串"=w270:string)  [unwired: 10 in]
            n184 = control-ref of="自定义起始时间"() -> (w286:refnum<vi>)
            n185 = control-ref of="自定义结束时间"() -> (w287:refnum<vi>)
            n186 = call "日期字符串格式至时间格式转换(子VI).vi"("data[0]"=w272) -> ("time stamp"=w277:timestamp)  [unwired: 10 in]
            n187 = call "日期字符串格式至时间格式转换(子VI).vi"("data[0]"=w270) -> ("time stamp"=w278:timestamp)  [unwired: 10 in]
            n188 = Bundle By Name(cluster=cluster{"起始范围":string, "截止范围":string} {"起始范围"="2", "截止范围"="5"} ("Single"), "起始范围"=w270, "截止范围"=w272) -> (w275:cluster{"起始范围":string, "截止范围":string})
            n189 = property class="XControl timepicker (严格)"(reference=w286, "Visible"=TRUE ("可见"), "Value"=w278) -> ()  [unwired: 1 in, 2 out]
            n190 = property class="XControl timepicker (严格)"(reference=w287, "Visible"=TRUE ("可见"), "Value"=w277) -> ()  [unwired: 1 in, 2 out]
            n191 = local write "自定义1single"(w275) -> ()
          }
        }
      }
      event "下拉列表": Value Change {
        w300 = FALSE ("可见")
        w290 = FALSE ("可见")
        n192 = event-data() -> ()  [unwired: 1 in, 6 out]
        n193 = local read "columns"() -> (w306:string[])
        n194 = control-ref of="自定义结束时间 2"() -> (w302:refnum<vi>)
        n195 = control-ref of="自定义起始时间 2"() -> (w301:refnum<vi>)
        n196 = control-ref of="自定义数值结束 2"() -> (w299:refnum<vi>)
        n197 = control-ref of="自定义数值起始 2"() -> (w292:refnum<vi>)
        n198 = control-ref of="自定义 2"() -> (w304:refnum<vi>)
        n199 = Search 1D Array(1D array=w306, element="下拉列表") -> (index of element=w308:i32)  [unwired: 1 in]
        n200 = property class="XControl timepicker (严格)"(reference=w302, "Visible"=w290) -> (error out=w297:errorcluster)  [unwired: 1 in, 1 out]
        n201 = property class="XControl timepicker (严格)"(reference=w301, "Visible"=w290) -> (error out=w296:errorcluster)  [unwired: 1 in, 1 out]
        n202 = property class="DigNum (严格)"(reference=w299, "Visible"=w300) -> (error out=w295:errorcluster)  [unwired: 1 in, 1 out]
        n203 = property class="DigNum (严格)"(reference=w292, "Visible"=w300) -> (error out=w294:errorcluster)  [unwired: 1 in, 1 out]
        n204 = property class="Clust (严格)"(reference=w304) -> (error out=w298:errorcluster, "Controls[]"=w303:refnum<vi>[])  [unwired: 1 in, 1 out]
        n205 = local read "type"() -> (w307:T3[])
        n206 = for {
          tunnel: w303 -> [w312] mode=indexing
          tunnel: [w310] -> _ mode=indexing
          n207 = property class="Ctl"(reference=w312, "Visible"=FALSE ("可见")) -> (reference out=w310:refnum<vi>)  [unwired: 1 in, 1 out]
        }
        n208 = Merge Errors(w298, w297, w296, w295, w294) -> (w293:errorcluster)
        n209 = Index Array(array=w307, index=w308) -> (element=w305:T3)
        n210 = control-ref of="标签 2"() -> (w291:refnum<vi>)
        n211 = case shown="\"String\", 默认" w305 {
          tunnel: "下拉列表" -> [w321 w354 w372]
          tunnel: w293 -> [_ _ _]
          tunnel: w291 -> [w317 w358 w378]
          frame "String", Default {
            n212 = property on="database" class="Str"() -> ("Value"=w313:string)  [unwired: 2 in, 2 out]
            n213 = property class="Str"(reference=w317, "Visible"=FALSE ("可见")) -> ()  [unwired: 1 in, 2 out]
            n214 = local read "table"() -> (w322:string)
            n215 = control-ref of="自定义 2"() -> (w319:refnum<vi>)
            n216 = call "查询clonm对应的所有内容.vi"("条件"=enum16{"DISTINCT", "MIN", "MAX"}."DISTINCT", "组合框"=w321, "database"=w313, "table"=w322) -> ("输出数组"=w320:string[])  [unwired: 6 in, 1 out]
            n217 = property class="Clust (严格)"(reference=w319) -> ("Controls[]"=w318:refnum<vi>[])  [unwired: 1 in, 2 out]
            n218 = call-poly <userlib>:"Remove Duplicates from 1D Array__ogtk.vi"("Input Array"=w320) -> ("Output Array"=w314:string[])  [unwired: 1 out]
            "自定义2筛选条件" <- w314
            n219 = for {
              tunnel: w314 -> [w324] mode=indexing
              tunnel: w318 -> [w325] mode=indexing
              n220 = case shown="\"lw\"" w324 {
                selector: w324 -> [w327 _ _ _ _ _ _ _ _ _ _ _ _ _ _ _ _ _]
                tunnel: [w327 "正常数据" "超上限" "超下限" "仪器故障" "仪器通信故障" "仪器离线" "维护调试数据" "缺试剂" "缺纯水" "缺水样" "缺标液" "加标回收" "平行样测试" "电源故障" "取水点无水样" "手工输入数据" "手动测试数据"] -> w323
                frame Default {
                }
                frame "N" {
                }
                frame "T" {
                }
                frame "L" {
                }
                frame "D" {
                }
                frame "F" {
                }
                frame "B" {
                }
                frame "M" {
                }
                frame "lr" {
                }
                frame "lp" {
                }
                frame "lw" {
                }
                frame "ls" {
                }
                frame "ra" {
                }
                frame "pt" {
                }
                frame "P" {
                }
                frame "Z" {
                }
                frame "S" {
                }
                frame "hd" {
                }
              }
              n221 = property class="Ctl"(reference=w325, "Caption.Text"=w323, "Visible"=TRUE ("可见")) -> ()  [unwired: 1 in, 2 out]
            }
          }
          frame "Long (I32)".."Double (DBL)" {
            w360 = TRUE ("可见")
            n222 = property on="database" class="Str"() -> ("Value"=w345:string)  [unwired: 2 in, 2 out]
            n223 = property class="Str"(reference=w358, "Visible"=TRUE ("可见")) -> ()  [unwired: 1 in, 2 out]
            n224 = local read "table"() -> (w355:string)
            n225 = call "查询clonm对应的所有内容.vi"("条件"=enum16{"DISTINCT", "MIN", "MAX"}."MAX", "组合框"=w354, "database"=w345, "table"=w355) -> ("输出数组"=w353:string[])  [unwired: 6 in, 1 out]
            n226 = call "查询clonm对应的所有内容.vi"("条件"=enum16{"DISTINCT", "MIN", "MAX"}."MIN", "组合框"=w354, "database"=w345, "table"=w355) -> ("输出数组"=w348:string[])  [unwired: 6 in, 1 out]
            n227 = Index Array(array=w353) -> (element=w346:string)  [unwired: 1 in]
            n228 = Index Array(array=w348) -> (element=w347:string)  [unwired: 1 in]
            n229 = control-ref of="自定义数值结束 2"() -> (w361:refnum<vi>)
            n230 = control-ref of="自定义数值起始 2"() -> (w362:refnum<vi>)
            n231 = Fract/Exp String To Number(string=w346) -> (number=w351:dbl)  [unwired: 3 in, 1 out]
            n232 = Fract/Exp String To Number(string=w347) -> (number=w352:dbl)  [unwired: 3 in, 1 out]
            n233 = Bundle By Name(cluster=cluster{"起始范围":string, "截止范围":string} {"起始范围"="2", "截止范围"="5"} ("Single"), "起始范围"=w347, "截止范围"=w346) -> (w350:cluster{"起始范围":string, "截止范围":string})
            n234 = property class="DigNum (严格)"(reference=w361, "Visible"=w360, "Value"=w351) -> ()  [unwired: 1 in, 2 out]
            n235 = property class="DigNum (严格)"(reference=w362, "Visible"=w360, "Value"=w352) -> ()  [unwired: 1 in, 2 out]
            n236 = local write "自定义2single"(w350) -> ()
          }
          frame "Date/Time" {
            n237 = property on="database" class="Str"() -> ("Value"=w363:string)  [unwired: 2 in, 2 out]
            n238 = property class="Str"(reference=w378, "Visible"=TRUE ("可见")) -> ()  [unwired: 1 in, 2 out]
            n239 = local read "table"() -> (w375:string)
            n240 = call "查询clonm对应的所有内容.vi"("条件"=enum16{"DISTINCT", "MIN", "MAX"}."MAX", "组合框"=w372, "database"=w363, "table"=w375) -> ("输出数组"=w374:string[])  [unwired: 6 in, 1 out]
            n241 = call "查询clonm对应的所有内容.vi"("条件"=enum16{"DISTINCT", "MIN", "MAX"}."MIN", "组合框"=w372, "database"=w363, "table"=w375) -> ("输出数组"=w373:string[])  [unwired: 6 in, 1 out]
            n242 = Index Array(array=w374) -> (element=w367:string)  [unwired: 1 in]
            n243 = Index Array(array=w373) -> (element=w365:string)  [unwired: 1 in]
            n244 = call "格式日期时间字符串.vi"("data[0]"=w367) -> ("日期/时间字符串"=w366:string)  [unwired: 10 in]
            n245 = call "格式日期时间字符串.vi"("data[0]"=w365) -> ("日期/时间字符串"=w364:string)  [unwired: 10 in]
            n246 = control-ref of="自定义起始时间 2"() -> (w380:refnum<vi>)
            n247 = control-ref of="自定义结束时间 2"() -> (w381:refnum<vi>)
            n248 = call "日期字符串格式至时间格式转换(子VI).vi"("data[0]"=w366) -> ("time stamp"=w371:timestamp)  [unwired: 10 in]
            n249 = call "日期字符串格式至时间格式转换(子VI).vi"("data[0]"=w364) -> ("time stamp"=w370:timestamp)  [unwired: 10 in]
            n250 = Bundle By Name(cluster=cluster{"起始范围":string, "截止范围":string} {"起始范围"="2", "截止范围"="5"} ("Single"), "起始范围"=w364, "截止范围"=w366) -> (w369:cluster{"起始范围":string, "截止范围":string})
            n251 = property class="XControl timepicker (严格)"(reference=w381, "Visible"=TRUE ("可见"), "Value"=w371) -> ()  [unwired: 1 in, 2 out]
            n252 = property class="XControl timepicker (严格)"(reference=w380, "Visible"=TRUE ("可见"), "Value"=w370) -> ()  [unwired: 1 in, 2 out]
            n253 = local write "自定义2single"(w369) -> ()
          }
        }
      }
      event "清空": Value Change {
        n254 = event-data() -> ()  [unwired: 1 in, 6 out]
        n255 = control-ref of="实时分钟小时数据"() -> (w387:refnum<vi>)
        n256 = control-ref of="下拉列表"() -> (w386:refnum<vi>)
        n257 = control-ref of="下拉列表 2"() -> (w385:refnum<vi>)
        n258 = control-ref of="测量模式"() -> (w391:refnum<vi>)
        n259 = control-ref of="自定义 2"() -> (w388:refnum<vi>)
        n260 = control-ref of="自定义"() -> (w389:refnum<vi>)
        n261 = Build Array(w386, w385) -> (w384:refnum<vi>[])
        n262 = Build Array(w391, w387, w388, w389) -> (w390:refnum<vi>[])
        n263 = for {
          tunnel: w384 -> [w392] mode=indexing
          n264 = invoke class="下拉列表 (严格)" method="Reinit To Default"(reference=w392) -> ()  [unwired: 2 in, 3 out]
        }
        n265 = for {
          tunnel: w390 -> [w393] mode=indexing
          n266 = invoke class="Clust" method="Reinit To Default"(reference=w393) -> ()  [unwired: 2 in, 3 out]
        }
      }
      event "确定": Value Change {
        w394 = TRUE
        n267 = event-data() -> ()  [unwired: 1 in, 6 out]
      }
      event "退出": Value Change; Panel Close {
        n268 = event-data() -> ()  [unwired: 1 in, 3 out]
      }
    }
  }
  "确定输出" <- w15
